vi "File_Array_2_Corr_Type.vi"(10 "Filenames IN":string[](array[string]), 11 "Extension":string) -> (3 "Only Filenames with Extension OUT":string[](array[string]))   [LabVIEW 2011]
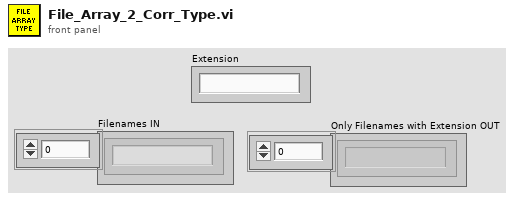
[diagram p1: front panel]
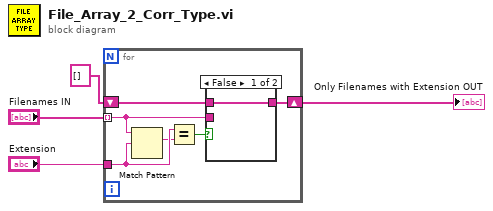
[diagram p0: block diagram]
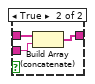
[diagram p2: hidden frame]
diagram:
  n1 = for {
    tunnel: "Filenames IN" -> [w8] mode=indexing
    shift-right: [w7] -> w4
    shift-left: string[] [] ("filenames") -> [w9]
    tunnel: "Extension" -> [w6]
    n2 = Match Pattern(string=w8, regular expression=w6) -> (match substring=w5:string)  [unwired: 1 in, 3 out]
    n3 = Equal?(x=w6, y=w5) -> (x = y?=w10:bool)
    n4 = case shown="False" w10 {
      tunnel: w9 -> [w11 w13]
      tunnel: w8 -> [_ w14]
      tunnel: [w11 w12] -> w7
      frame False {
      }
      frame True {
        n5 = Build Array (concatenate)(w13, w14) -> (w12:string[])
      }
    }
  }
  "Only Filenames with Extension OUT" <- w4
